vi "시리얼_읽기.vi"(8 "Error In":errorcluster caption="에러 입력", 10 "바이트 카운트":u32, 11 "VISA 리소스 이름":refnum<visa-resource-name>) -> (0 "Error Out":errorcluster caption="에러 출력", 1 "반환 카운트":u32, 2 "Resoponse":string, 3 "VISA 리소스 이름 출력":refnum<visa-resource-name>)   [LabVIEW 2015]
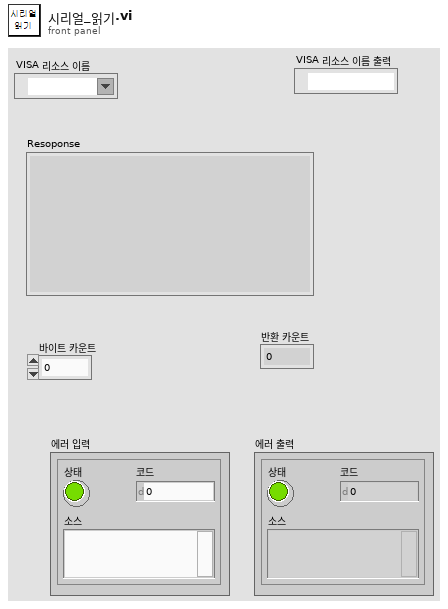
[diagram p1: front panel]
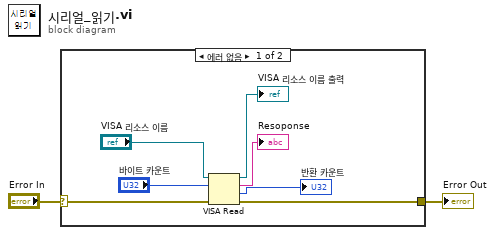
[diagram p0: block diagram]
diagram:
  n1 = case shown="에러 없음" "Error In" {
    selector: "Error In" -> [w9 w10]
    tunnel: [w8 w10] -> w1
    frame No Error {
      n2 = VISA Read(VISA resource name="VISA 리소스 이름", byte count="바이트 카운트", error in (no error)=w9) -> (VISA resource name out=→"VISA 리소스 이름 출력":refnum<visa-resource-name>, read buffer=→"Resoponse":string, return count=→"반환 카운트":u32, error out=w8:errorcluster)
    }
    frame Error {
    }
  }
  "Error Out" <- w1
